vi "量测结果提取.vi"(0 "量测信息":T7[](array[typedef]), 5 "相机1":T6[](array[typedef]), 7 "相机2":T6[](array[typedef]), 9 "当前出料信息":T5, 11 "ModelEditInfo":T1={"Root"=path "", "AllModelFold"=path "", "AllModelNamePath"=path "", "所有零件型号"=[], "当前零件型号"="", "所有建立零件信息"=[], "当前零件序号"=0, "当前量测项目序号"=0, "当前量测零件信息"={"所有量测项目"=[], "相机1量测项目"=[], "相机2量测项目"=[], "相机3量测项目"=[], "相机是否使用"=[], "当前量测程式路径Cam1"=path "", "当前量测程式路径Cam2"=path "", "当前量测程式路径Cam3"=path "", "当前量测项路径"=path "", "4只相机量测规格"={"相机1量测规格"=[], "相机2量测规格"=[], "相机3量测规格"=[], "相机4量测规格"=[]}, "相机4量测项目"=[], "当前量测程式路径Cam4"=path "", "4只相机校正比例"={"相机1校正比例"=[], "相机2校正比例"=[], "相机3校正比例"=[], "相机4校正比例"=[]}, "拍照间隔时间"={"入料感应与Cam1时间S"=5.0, "入料感应与Cam2时间S"=10.0, "入料感应与Cam3时间S"=15.0, "出料感应与卸料时间S"=0.0}, "报警不良数"=0}} {"当前量测零件信息"."4只相机量测规格"."相机4量测规格"."上限" format="%#.4g"; "当前量测零件信息"."4只相机量测规格"."相机4量测规格"."下限" format="%#.4g"; "当前量测零件信息"."4只相机量测规格"."相机3量测规格"."上限" format="%#.4g"; "当前量测零件信息"."4只相机量测规格"."相机3量测规格"."下限" format="%#.4g"; "当前量测零件信息"."4只相机量测规格"."相机2量测规格"."上限" format="%#.4g"; "当前量测零件信息"."4只相机量测规格"."相机2量测规格"."下限" format="%#.4g"; "当前量测零件信息"."4只相机量测规格"."相机1量测规格"."上限" format="%#.4g"; "当前量测零件信息"."4只相机量测规格"."相机1量测规格"."下限" format="%#.4g"}) -> (4 "有量测完成":bool, 6 "量测结果":bool, 10 "当前出料信息":T5)   [LabVIEW 2014]
uses:
  Controls/TestThreshold.ctl
  ModelEditSubVIs/ModeEditeControl.ctl
panel:
  # "~"
  # "~"
  # "~"
  # "~"
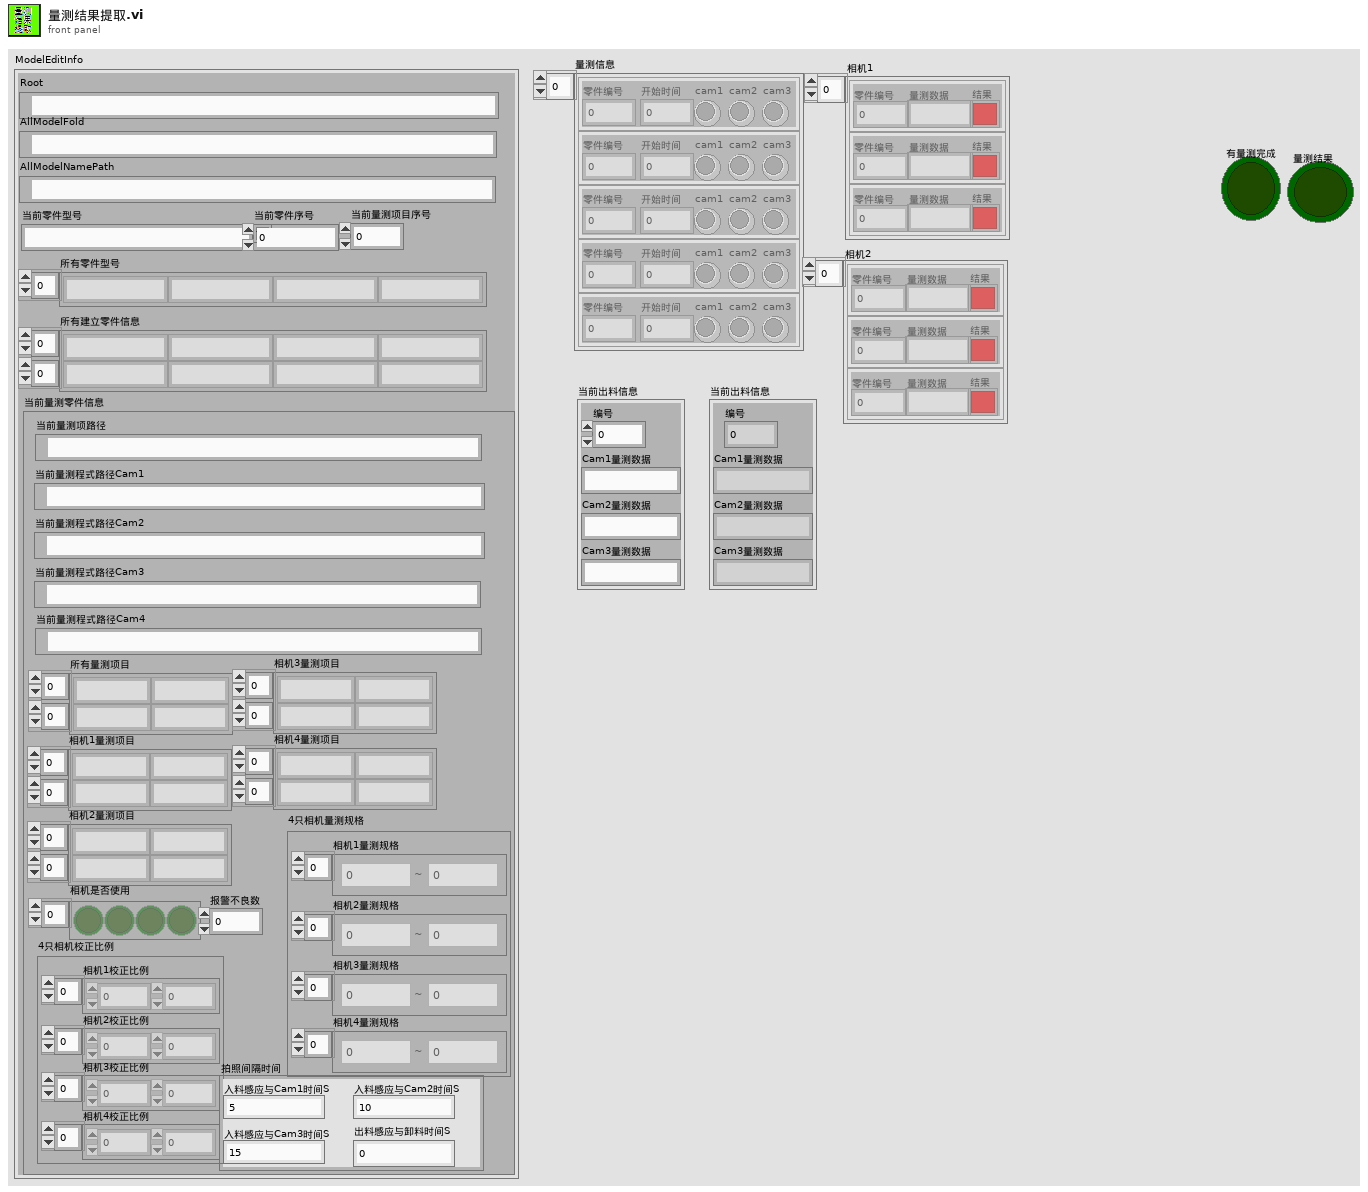
[diagram p1: front panel]
types:
  T1 = typedef "ModeEditeControl.ctl" = cluster{"Root":path, "AllModelFold":path, "AllModelNamePath":path, "所有零件型号":string[], "当前零件型号":string, "所有建立零件信息":string[][], "当前零件序号":i32, "当前量测项目序号":i32, "当前量测零件信息":cluster{"所有量测项目":string[][], "相机1量测项目":string[][], "相机2量测项目":string[][], "相机3量测项目":string[][], "相机是否使用":bool[], "当前量测程式路径Cam1":path, "当前量测程式路径Cam2":path, "当前量测程式路径Cam3":path, "当前量测项路径":path, "4只相机量测规格":T2, "相机4量测项目":string[][], "当前量测程式路径Cam4":path, "4只相机校正比例":cluster{"相机1校正比例":dbl[], "相机2校正比例":dbl[], "相机3校正比例":dbl[], "相机4校正比例":dbl[]}, "拍照间隔时间":T4, "报警不良数":i32}}
  T2 = typedef "4只相机量测规格.ctl" = cluster{"相机1量测规格":T3[], "相机2量测规格":T3[], "相机3量测规格":T3[], "相机4量测规格":T3[]}
  T3 = typedef "TestThreshold.ctl" = cluster{"下限":dbl, "上限":dbl}
  T4 = typedef "拍照间隔时间设定.ctl" = cluster{"入料感应与Cam1时间S":dbl, "入料感应与Cam2时间S":dbl, "入料感应与Cam3时间S":dbl, "出料感应与卸料时间S":dbl}
  T5 = typedef "当前出料信息.ctl" = cluster{"编号":i64, "Cam1量测数据":string, "Cam2量测数据":string, "Cam3量测数据":string}
  T6 = typedef "量测结果.ctl" = cluster{"量测数据":string, "结果":bool, "零件编号":dbl}
  T7 = typedef "工件信息.ctl" = cluster{"零件编号":i64, "开始时间":i64, "cam1":bool, "cam2":bool, "cam3":bool}
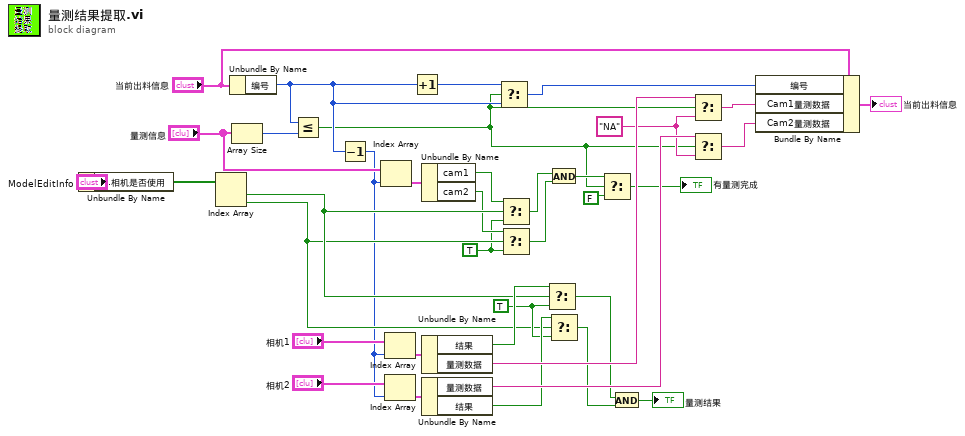
[diagram p0: block diagram]
diagram:
  w3 = TRUE ("f")
  w10 = TRUE ("f")
  w20 = "NA"
  n1 = Unbundle By Name("ModelEditInfo") -> ("当前量测零件信息.相机是否使用"=w15:bool[])
  n2 = Index Array(array=w15) -> (element #1=w9:bool, element #2=w6:bool)  [unwired: 2 in]
  n3 = Unbundle By Name("当前出料信息") -> ("编号"=w26:i64)
  n4 = Array Size(array="量测信息") -> (size(s)=w28:i32)
  n5 = Less Or Equal?(x=w26, y=w28) -> (x <= y?=w2:bool)
  n6 = Decrement(x=w26) -> (x-1=w1:i64)
  n7 = Index Array(array="量测信息", index=w1) -> (element=w33:T7)
  n8 = Index Array(array="相机1", index=w1) -> (element=w35:T6)
  n9 = Index Array(array="相机2", index=w1) -> (element=w34:T6)
  n10 = Increment(x=w26) -> (x+1=w27:i64)
  n11 = Unbundle By Name(w33) -> ("cam1"=w8:bool, "cam2"=w5:bool)
  n12 = Unbundle By Name(w35) -> ("结果"=w14:bool, "量测数据"=w24:string)
  n13 = Unbundle By Name(w34) -> ("量测数据"=w22:string, "结果"=w12:bool)
  n14 = Select(t=w27, s=w2, f=w26) -> (s? t:f=w25:i64)
  n15 = Select(t=w8, s=w9, f=w3) -> (s? t:f=w7:bool)
  n16 = Select(t=w5, s=w6, f=w3) -> (s? t:f=w4:bool)
  n17 = Select(t=w14, s=w9, f=w10) -> (s? t:f=w13:bool)
  n18 = And(x=w7, y=w4) -> (x .and. y?=w19:bool)
  n19 = Select(t=w12, s=w6, f=w10) -> (s? t:f=w11:bool)
  n20 = Select(t=w19, s=w2, f=FALSE) -> (s? t:f=→"有量测完成":bool)
  n21 = And(x=w13, y=w11) -> (x .and. y?=→"量测结果":bool)
  n22 = Select(t=w24, s=w2, f=w20) -> (s? t:f=w23:string)
  n23 = Select(t=w22, s=w2, f=w20) -> (s? t:f=w21:string)
  n24 = Bundle By Name(cluster="当前出料信息", "编号"=w25, "Cam1量测数据"=w23, "Cam2量测数据"=w21) -> (→"当前出料信息":T5)
